vi "ConfigureTestPanel.vi"(8 "error in (no error)":errorcluster) -> (0 "error out":errorcluster, 2 "DataGroups ChannelStatus":T1[](array[typedef]), 3 "Test Panel Config out":T3)   [LabVIEW 2017, in "McsaTestPanel.lvlib"]
uses:
  <vilib>/addons/InsightCM/Devices/Shared/Mcsa/McsaTestPanel/McsaTestPanel.lvlib
  <vilib>/addons/InsightCM/Devices/Shared/Mcsa/McsaTestPanel/controls/Configuration.ctl
  <vilib>/addons/InsightCM/Devices/Shared/Common/TestPanel/controls/Configuration.ctl
  <vilib>/addons/InsightCM/Devices/Shared/Common/TestPanel/controls/State.ctl
  <vilib>/addons/InsightCM/MessageBus/Base/controls/IRoutingSource.ctl
  <vilib>/addons/InsightCM/Devices/Shared/Mcsa/McsaTestPanel/controls/ChannelStatus.ctl
  <vilib>/addons/InsightCM/MessageBus/Base/controls/KeyValuePair.ctl
  <vilib>/addons/InsightCM/MessageBus/Base/controls/TestPanelTimeSeries.ctl
  <vilib>/addons/InsightCM/MessageBus/Base/controls/TestPanelValue.ctl
  <vilib>/addons/InsightCM/Devices/Shared/Common/TestPanel/TestPanel.lvlib
  <vilib>/addons/InsightCM/Utilities/DeviceModelHelpers/DeviceModelHelpers.lvlib
  <vilib>/addons/InsightCM/Utilities/GlobalConfiguration/GlobalConfiguration.lvlib
  <vilib>/addons/InsightCM/Utilities/PropertyHelpers/PropertyHelpers.lvlib
  <vilib>/addons/InsightCM/Devices/Shared/Mcsa/McsaVirtualChannel/McsaVirtualChannel.lvlib
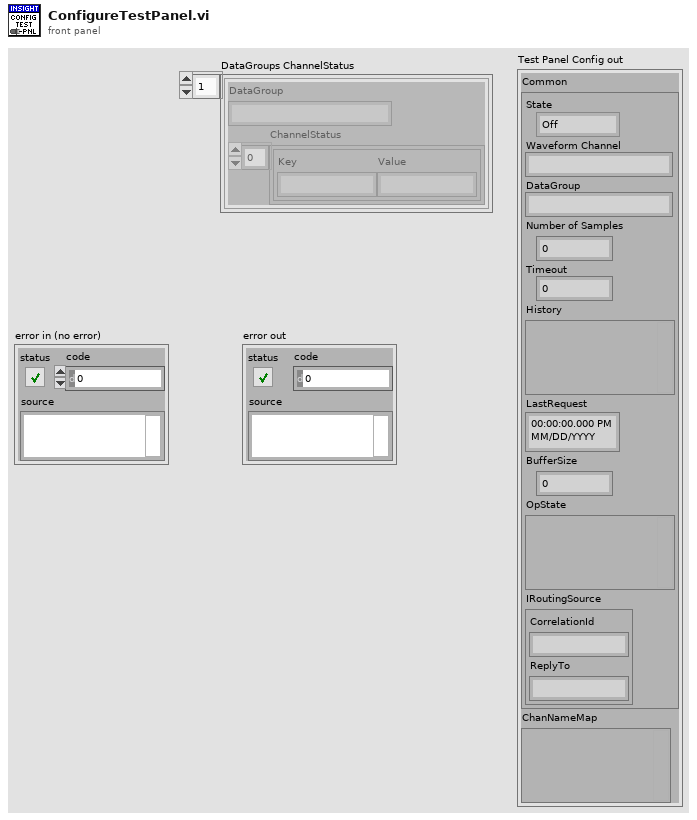
[diagram p1: front panel]
types:
  T1 = typedef "McsaTestPanel.lvlib/ChannelStatus.ctl" = cluster{"DataGroup":string, "ChannelStatus":T2[]}
  T2 = typedef "KeyValuePair.ctl" = cluster{"Key":string, "Value":string}
  T3 = typedef "McsaTestPanel.lvlib/Configuration.ctl" = cluster{"Common":T4, "ChanNameMap":variant}
  T4 = typedef "TestPanel.lvlib/Configuration.ctl" = cluster{"State":T5, "Waveform Channel":string, "DataGroup":string, "Number of Samples":i32, "Timeout":dbl, "History":variant, "LastRequest":timestamp, "BufferSize":i32, "OpState":variant, "IRoutingSource":T6}
  T5 = typedef "TestPanel.lvlib/State.ctl" = enum16{"Off", "On", "PendingValues", "PendingDataSet"}
  T6 = typedef "IRoutingSource.ctl" = cluster{"CorrelationId":string, "ReplyTo":string}
  T7 = typedef "SectionKeyValues.ctl" = cluster{"Section":string, "KeyValues":T2[]}
  T8 = typedef "R2_Channel.ctl" = cluster{"Id":string, "DeviceId":string, "Name":string, "ChannelType":string, "HardwareKey":string, "HardwareChannel":string, "DataGroup":string, "Keywords":string[], "EquipmentIds":string[], "Properties":T2[], "Metrics":T9[], "AssetNodeId":string, "MeasType":string, "AssetName":string}
  T9 = typedef "Metric.ctl" = cluster{"Id":string, "Name":string, "Unit":string, "Properties":T2[], "MetricDefinitionInstanceId":string}
  T10 = typedef "AssetNode.ctl" = cluster{"Id":string, "Type":string, "Name":string, "ParentIds":string[], "State":T11, "MeasType":string, "Properties":T2[], "OperatingStates":T12[], "Metrics":T9[], "TrendAlarmRules":T15[], "References":T18[]}
  T11 = typedef "AssetState.ctl" = cluster{"Disabled":bool}
  T12 = typedef "OperatingState.ctl" = cluster{"Name":string, "Properties":T2[], "Triggers":T13[]}
  T13 = typedef "Trigger.ctl" = cluster{"Type":string, "Expression":string, "Conditions":T14[]}
  T14 = typedef "Condition.ctl" = cluster{"Source":string, "Type":string, "Operator":string, "CompareTo":string, "DwellSeconds":dbl}
  T15 = typedef "TrendAlarmRule.ctl" = cluster{"Id":string, "AssetNodeId":string, "TrendId":string, "Disabled":bool, "OperatingState":string, "Operator":string, "Hysteresis":dbl, "OnDelaySeconds":dbl, "OffDelaySeconds":dbl, "Levels":T16[], "Properties":T2[]}
  T16 = typedef "TrendAlarmLevel.ctl" = cluster{"Severity":i32, "CompareTo":dbl, "Actions":T17[]}
  T17 = typedef "AlarmAction.ctl" = cluster{"Type":string, "Props":T2[]}
  T18 = typedef "AssetNodeReference.ctl" = cluster{"NodeId":string, "Name":string}
  T19 = typedef "TestPanelTimeSeries.ctl" = cluster{"TrendPointId":string, "AssetName":string, "MetricName":string, "Unit":string, "Values":T20[]}
  T20 = typedef "TestPanelValue.ctl" = cluster{"Value":dbl, "Timestamp":i64, "Invalid":bool}
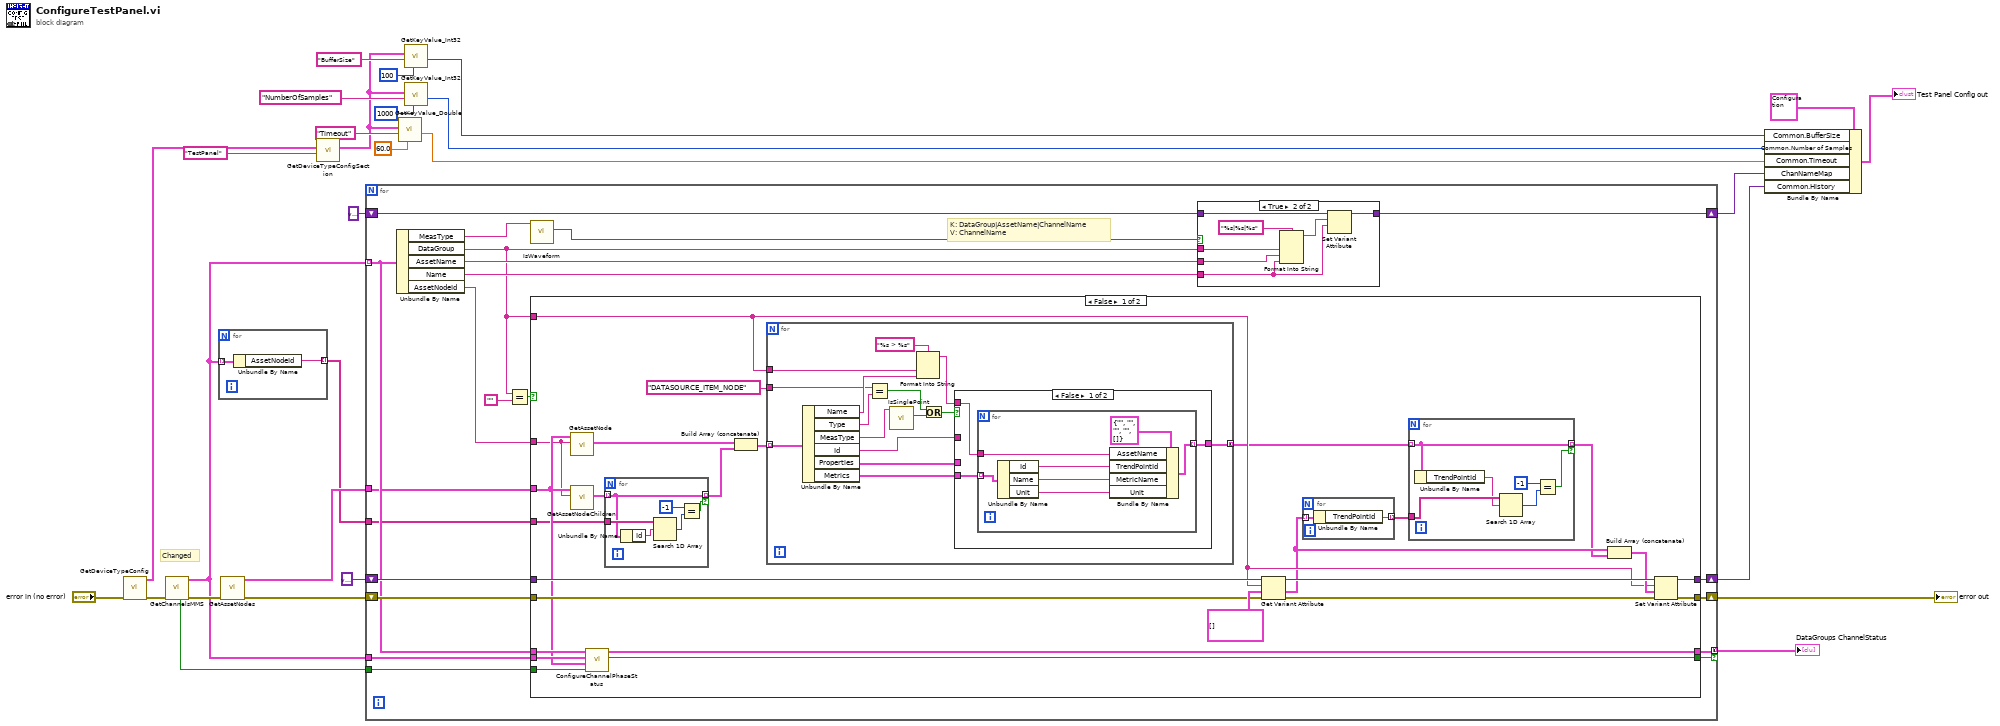
[diagram p0: block diagram]
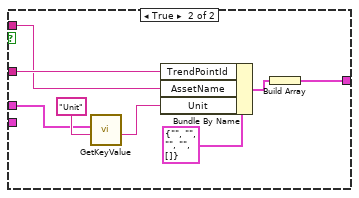
[diagram p3: hidden frame]
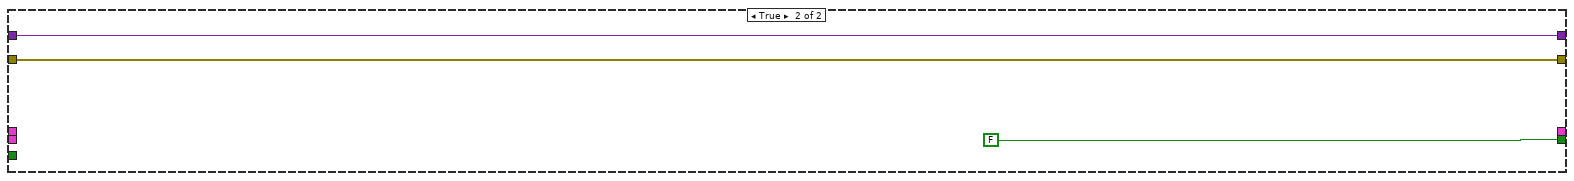
[diagram p4: hidden frame]
diagram:
  # "Changed"
  n1 = call <vilib>:"GetDeviceTypeConfig.vi"("error in (no error)"="error in (no error)") -> ("error out"=w9:errorcluster, "key values"=w25:T7[])  [unwired: 8 in, 1 out]
  n2 = call <vilib>:"GetChannelsMMS.vi"("error in (no error)"=w9) -> ("error out"=w8:errorcluster, "MMS Channels"=w2:T8[], "shared data group exists?"=w7:bool)  [unwired: 6 in, 2 out]
  n3 = for {
    tunnel: w2 -> [w30] mode=indexing
    tunnel: [w29] -> w1 mode=indexing
    n4 = Unbundle By Name(w30) -> ("AssetNodeId"=w29:string)
  }
  n5 = call <vilib>:"GetAssetNodes.vi"("error in (no error)"=w8) -> ("error out"=w15:errorcluster, "AssetNodes"=w27:T10[])  [unwired: 8 in, 1 out]
  n6 = call <vilib>:"GetDeviceTypeConfigSection.vi"("key"="TestPanel", "key values"=w25) -> ("key value pairs out"=w12:T2[])  [unwired: 8 in, 1 out]
  n7 = for {
    tunnel: w2 -> [w46] mode=indexing
    tunnel: w27 -> [w44]
    shift-right: [w49] -> w17
    shift-left: variant -> [w50]
    shift-right: [w48] -> w16
    shift-left: w15 -> [w47]
    tunnel: w2 -> [w45]
    tunnel: w7 -> [w41]
    shift-right: [w35] -> w6
    shift-left: variant -> [w34]
    tunnel: [w33] -> w4 mode=concatenating if=w32
    tunnel: w1 -> [w31]
    # "K: DataGroup|AssetName|ChannelName\nV: ChannelName"
    n8 = Unbundle By Name(w46) -> ("MeasType"=w37:string, "DataGroup"=w38:string, "AssetName"=w39:string, "Name"=w40:string, "AssetNodeId"=w51:string)
    n9 = Equal?(x=w38, y="") -> (x = y?=w42:bool)
    n10 = call <vilib>:"IsWaveform.vi"("MeasType"=w37) -> ("is waveform"=w36:bool)  [unwired: 10 in]
    n11 = case shown="False" w42 {
      tunnel: w51 -> [w67 _]
      tunnel: w50 -> [w85 w135]
      tunnel: w38 -> [w71 _]
      tunnel: [w81 w135] -> w49
      tunnel: [w79 w134] -> w48
      tunnel: w47 -> [w78 w134]
      tunnel: w46 -> [w70 _]
      tunnel: w45 -> [w74 _]
      tunnel: w44 -> [w68 _]
      tunnel: [w73 _] -> w33
      tunnel: [w69 FALSE ("valid?")] -> w32
      tunnel: w41 -> [w72 _]
      tunnel: w31 -> [w66 _]
      frame False {
        n12 = call <vilib>:"GetAssetNode.vi"("node id"=w67, "nodes in"=w68) -> ("AssetNode"=w76:T10)  [unwired: 7 in, 2 out]
        n13 = call <vilib>:"GetAssetNodeChildren.vi"("node id"=w67, "nodes in"=w68) -> ("Children"=w64:T10[])  [unwired: 8 in, 1 out]
        n14 = call <vilib>:"ConfigureChannelPhaseStatus.vi"("shared data group exist?"=w72, "AssetNodes"=w68, "AllChannels"=w74, "ChannelModel"=w70) -> ("valid"=w69:bool, "DataGroup ChannelStatus Out"=w73:T1[])  [unwired: 6 in]
        n15 = for {
          tunnel: w64 -> [w96] mode=indexing
          tunnel: w66 -> [w98]
          tunnel: [w96] -> w65 mode=indexing if=w94
          n16 = Unbundle By Name(w96) -> ("Id"=w99:string)
          n17 = Search 1D Array(1D array=w98, element=w99) -> (index of element=w97:i32)  [unwired: 1 in]
          n18 = Equal?(x=-1, y=w97) -> (x = y?=w94:bool)
        }
        n19 = Build Array (concatenate)(w76, w65) -> (w75:T10[])
        n20 = for {
          tunnel: w75 -> [w102] mode=indexing
          tunnel: [w103] -> w61 mode=concatenating
          tunnel: "DATASOURCE_ITEM_NODE" ("x") -> [w101]
          tunnel: w71 -> [w100]
          n21 = Unbundle By Name(w102) -> ("Name"=w105:string, "Type"=w111:string, "MeasType"=w112:string, "Id"=w114:string, "Properties"=w107:T2[], "Metrics"=w113:T9[])
          n22 = Equal?(x=w101, y=w111) -> (x = y?=w108:bool)
          n23 = call <vilib>:"IsSinglePoint.vi"("MeasType"=w112) -> ("is single point"=w110:bool)  [unwired: 10 in]
          n24 = Format Into String(format string="%s > %s", w100, w105) -> (resulting string=w104:string)  [unwired: 2 in, 1 out]
          n25 = Or(x=w108, y=w110) -> (x .or. y?=w109:bool)
          n26 = case shown="False" w109 {
            tunnel: w114 -> [_ w131]
            tunnel: [w116 w129] -> w103
            tunnel: w113 -> [w117 _]
            tunnel: w107 -> [_ w127]
            tunnel: w104 -> [w115 w125]
            frame False {
              n27 = for {
                tunnel: w117 -> [w123] mode=indexing
                tunnel: [w121] -> w116 mode=indexing
                tunnel: w115 -> [w120]
                n28 = Unbundle By Name(w123) -> ("Id"=w122:string, "Name"=w119:string, "Unit"=w118:string)
                n29 = Bundle By Name(cluster=T19 {"TrendPointId"="", "AssetName"="", "MetricName"="", "Unit"="", "Values"=[]} ("History"), "AssetName"=w120, "TrendPointId"=w122, "MetricName"=w119, "Unit"=w118) -> (w121:T19)
              }
            }
            frame True {
              n30 = call <vilib>:"GetKeyValue.vi"("key"="Unit" ("name"), "key value pairs"=w127) -> ("value"=w126:string)  [unwired: 7 in, 2 out]
              n31 = Bundle By Name(cluster=T19 {"TrendPointId"="", "AssetName"="", "MetricName"="", "Unit"="", "Values"=[]} ("History"), "TrendPointId"=w131, "AssetName"=w125, "Unit"=w126) -> (w130:T19)
              n32 = Build Array(w130) -> (w129:T19[])
            }
          }
        }
        n33 = Get Variant Attribute(Variant=w85, name=w71, default value (empty Variant)=T19[] [], error in=w78) -> (duplicate Variant=w83:variant, value=w63:T19[], error out=w80:errorcluster)  [unwired: 1 out]
        n34 = for {
          tunnel: w63 -> [w93] mode=indexing
          tunnel: [w92] -> w62 mode=indexing
          n35 = Unbundle By Name(w93) -> ("TrendPointId"=w92:string)
        }
        n36 = for {
          tunnel: w62 -> [w91]
          tunnel: w61 -> [w87] mode=indexing
          tunnel: [w87] -> w60 mode=indexing if=w86
          n37 = Unbundle By Name(w87) -> ("TrendPointId"=w90:string)
          n38 = Search 1D Array(1D array=w91, element=w90) -> (index of element=w88:i32)  [unwired: 1 in]
          n39 = Equal?(x=-1, y=w88) -> (x = y?=w86:bool)
        }
        n40 = Build Array (concatenate)(w63, w60) -> (w82:T19[])
        n41 = Set Variant Attribute(Variant=w83, name=w71, value=w82, error in=w80) -> (Variant out=w81:variant, error out=w79:errorcluster)  [unwired: 1 out]
      }
      frame True {
      }
    }
    n42 = case shown="True" w36 {
      tunnel: w34 -> [w52 w59]
      tunnel: [w52 w58] -> w35
      tunnel: w38 -> [_ w56]
      tunnel: w39 -> [_ w54]
      tunnel: w40 -> [_ w53]
      frame False {
      }
      frame True {
        n43 = Format Into String(format string="%s|%s|%s", w56, w54, w53) -> (resulting string=w55:string)  [unwired: 2 in, 1 out]
        n44 = Set Variant Attribute(Variant=w59, name=w55, value=w53) -> (Variant out=w58:variant)  [unwired: 1 in, 2 out]
      }
    }
  }
  "error out" <- w16
  "DataGroups ChannelStatus" <- w4
  n45 = call <vilib>:"GetKeyValue_Double.vi"("default"=60.0, "key"="Timeout", "key value pairs"=w12) -> ("value"=w19:dbl)  [unwired: 6 in, 2 out]
  n46 = call <vilib>:"GetKeyValue_Int32.vi"("default"=100, "key"="BufferSize", "key value pairs"=w12) -> ("value"=w10:i32)  [unwired: 6 in, 2 out]
  n47 = call <vilib>:"GetKeyValue_Int32.vi"("default"=1000, "key"="NumberOfSamples", "key value pairs"=w12) -> ("value"=w18:i32)  [unwired: 6 in, 2 out]
  n48 = Bundle By Name(cluster=T3 {"Common"={"State"=enum."Off", "Waveform Channel"="", "DataGroup"="", "Number of Samples"=0, "Timeout"=0.0, "History"=variant, "LastRequest"=timestamp(0 s since 1904-01-01), "BufferSize"=0, "OpState"=variant, "IRoutingSource"={"CorrelationId"="", "ReplyTo"=""}}, "ChanNameMap"=variant} ("Test Panel Config out 2"), "Common.BufferSize"=w10, "Common.Number of Samples"=w18, "Common.Timeout"=w19, "ChanNameMap"=w6, "Common.History"=w17) -> (→"Test Panel Config out":T3)
